vi "DMA Error Global.vi"(2 "Write (F)":bool, 7 "Error In":bool) -> (8 "Error Out":bool)   [LabVIEW 2019]
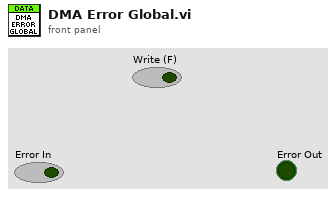
[diagram p1: front panel]
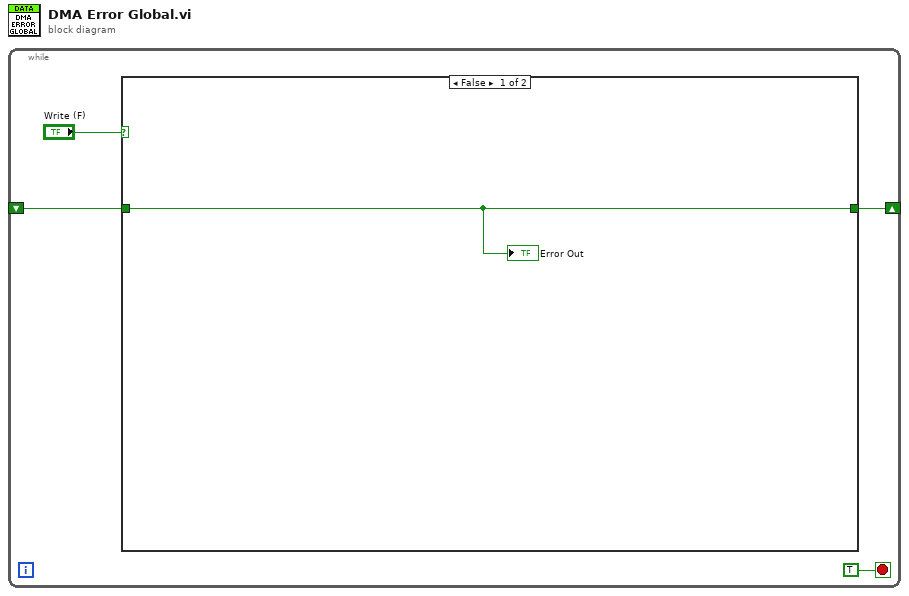
[diagram p0: block diagram]
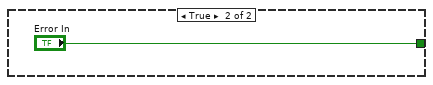
[diagram p2: hidden frame]
diagram:
  n1 = while {
    shift-right: [w2] -> _
    shift-left: _ -> [w1]
    stop <- TRUE stop-if-true
    n2 = case shown="False" "Write (F)" {
      tunnel: [w5 "Error In"] -> w2
      tunnel: w1 -> [w5 _]
      frame False {
        "Error Out" <- w5
      }
      frame True {
      }
    }
  }
